vi "Timer_Reset.vi"(11 "in TIMER":T1 {"Accumulated TIme" format="%13.5p"; "StartTime" format="%13.5p"}) -> (3 "out TIMER":T1 {"Accumulated TIme" format="%13.5p"; "StartTime" format="%13.5p"})   [LabVIEW 2019, in "Trajectory_Library.lvlib"]
doc: "Reset the timer by setting the time to 0. Make the timer startTime the current time so new requests will be relative now\n\nInputs:\n - Timer -- The Timer data cluster\n\nOutputs:\n - Timer -- The modified Timer data cluster"
uses:
  Trajectory_Library.lvlib
  TIMER.ctl
  Util_GetTime.vi
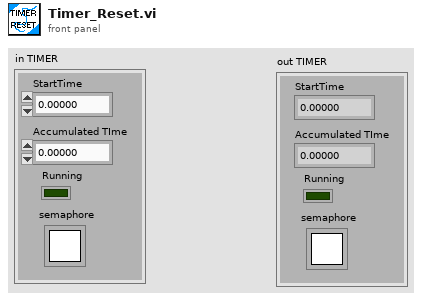
[diagram p1: front panel]
types:
  T1 = typedef "Trajectory_Library.lvlib/TIMER.ctl" = cluster{"StartTime":dbl, "Accumulated TIme":dbl, "Running":bool, "semaphore":T2}
  T2 = typedef "Semaphore RefNum" = refnum<k1>
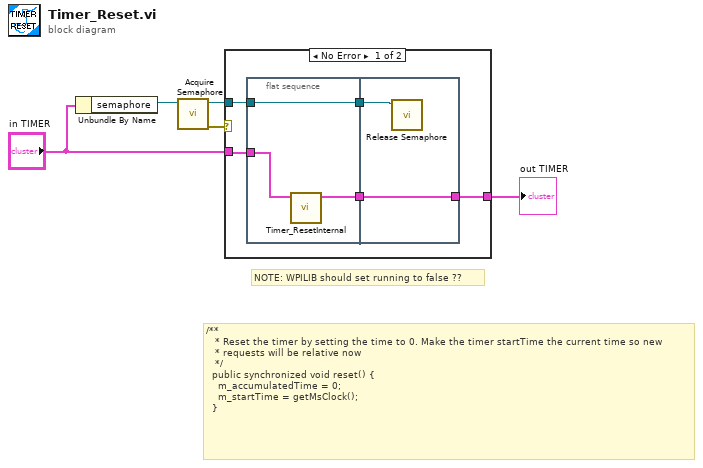
[diagram p0: block diagram]
diagram:
  # "NOTE: WPILIB should set running to false ??"
  # "/**\n   * Reset the timer by setting the time to 0. Make the timer startTime the current time so new\n   * requests will be relative now\n   */\n  public synchronized void reset() {\n    m_accumulatedTime = 0;\n    m_startTime = getMsClock();\n  }"
  n1 = Unbundle By Name("in TIMER") -> ("semaphore"=w4:T2)
  n2 = call <vilib>:"Acquire Semaphore.vi"("semaphore"=w4) -> ("error out"=w3:errorcluster, "semaphore out"=w1:T2)  [unwired: 4 in, 1 out]
  n3 = case shown="No Error" w3 {
    tunnel: [w10 w16] -> w5
    tunnel: "in TIMER" -> [w9 w16]
    tunnel: w1 -> [w6 _]
    frame No Error {
      n4 = flat-sequence {
        tunnel: w9 -> [w12]
        tunnel: [w13] -> w8
        tunnel: [w11] -> w7
        tunnel: w6 -> [w11]
        tunnel: [w15] -> w10
        tunnel: w8 -> [w15]
        tunnel: w7 -> [w14]
        frame #0 {
          n5 = call "Timer_ResetInternal.vi"("in TIMER"=w12) -> ("out TIMER"=w13:T1)  [unwired: 10 in]
        }
        frame #1 {
          n6 = call <vilib>:"Release Semaphore.vi"("semaphore"=w14) -> ()  [unwired: 5 in, 2 out]
        }
      }
    }
    frame Error {
    }
  }
  "out TIMER" <- w5
